vi "MakeProfileMovies.vi"(6 "Plot Metadata":T1[](array[typedef]), 7 "Job Directory":path, 9 "templatePath":path, 10 "Result files to read":path[](array[path]), 11 "suggestedName":string) -> (0 "error out":errorcluster, 3 "automaticFilename":string)   [LabVIEW 2021]
uses:
  Anemometry/Anemometry Sub Vis/Data_plotting_vis/RFP_Plot_Metadata.ctl
  Anemometry/Anemometry Sub Vis/Data_plotting_vis/Error_bars_index.ctl
panel:
  in  "Stop":bool
  out "ffmpegOutput":string
  # "Harvests images corresponding to Raw Data files of plotted series. Joins multiple cam images per measurement, and joins those alongside joined images from other series"
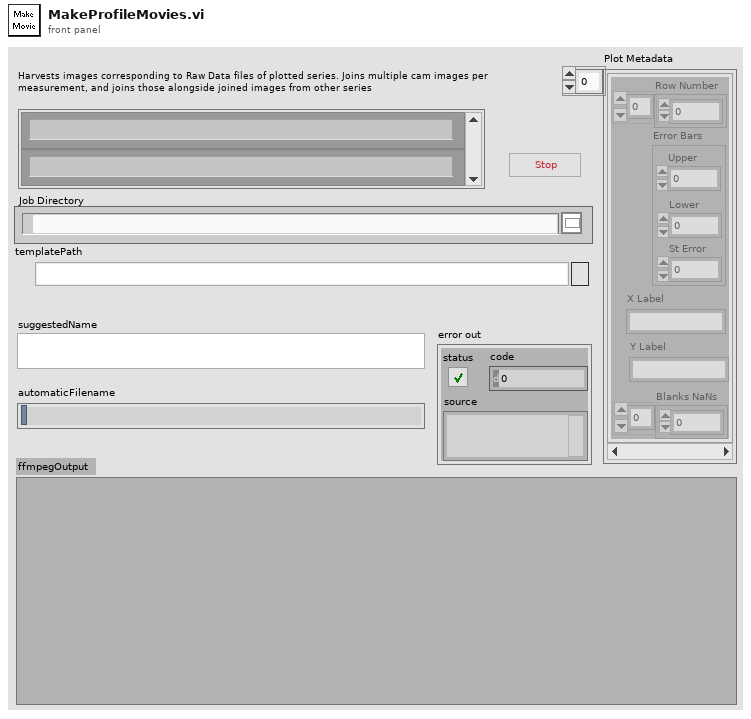
[diagram p1: front panel]
types:
  T1 = typedef "RFP_Plot_Metadata.ctl" = cluster{"Row Number":i32[], "Error Bars":T2, "X Label":string, "Y Label":string, "Blanks NaNs":i32[]}
  T2 = typedef "Error_bars_index.ctl" = cluster{"Upper":i32, "Lower":i32, "St Error":i32}
  T3 = cluster{"new picture":picture, "image path":path}[]
  T4 = typedef "imagedata.ctl" = cluster{"image type":i32, "image depth":i32, "image":u8[], "mask":u8[], "colors":u32[], "Rectangle":cluster{"left":i16, "top":i16, "right":i16, "bottom":i16}}
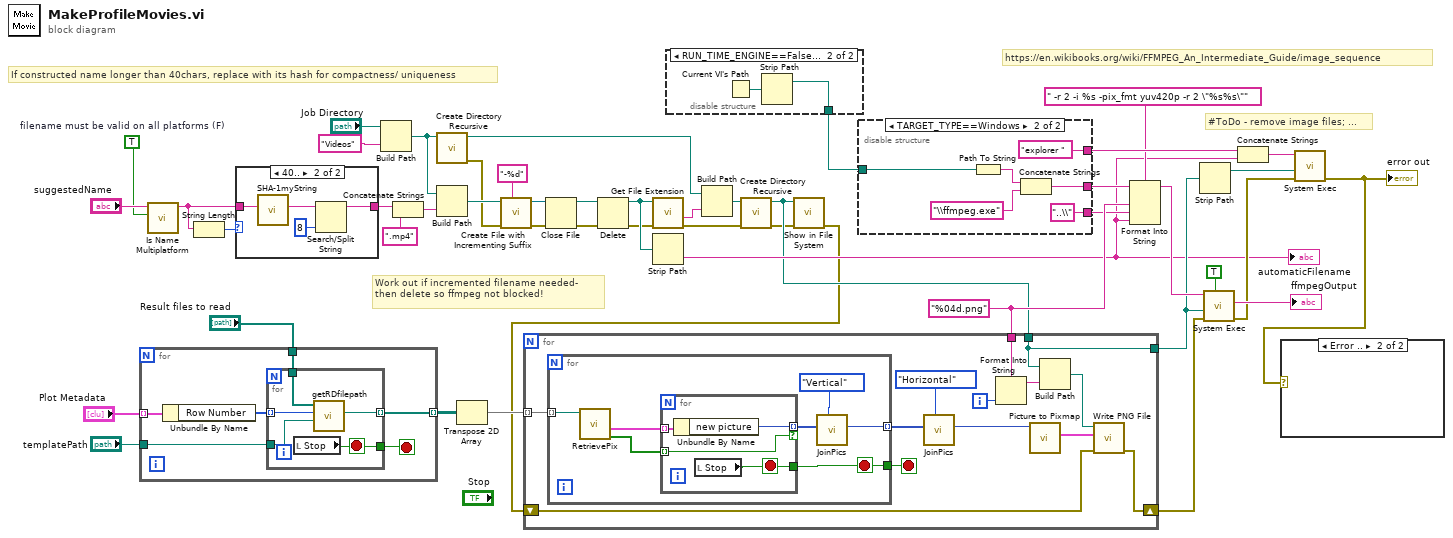
[diagram p0: block diagram]
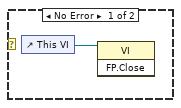
[diagram p2: hidden frame]
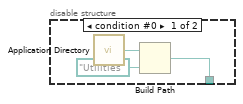
[diagram p3: hidden frame]
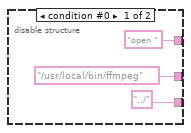
[diagram p5: hidden frame]
diagram:
  w38 = TRUE  # filename must be valid on all platforms (F)
  w27 = "%04d.png" ("format string")
  # "Work out if incremented filename needed- then delete so ffmpeg not blocked!"
  # "If constructed name longer than 40chars, replace with its hash for compactness/ uniqueness"
  # "#ToDo - remove image files; ..."
  # "https://en.wikibooks.org/wiki/FFMPEG_An_Intermediate_Guide/image_sequence"
  n1 = for {
    tunnel: "Plot Metadata" -> [w53] mode=indexing
    tunnel: [w50] -> w45 mode=indexing
    tunnel: "Result files to read" -> [w51]
    tunnel: "templatePath" -> [w49]
    stop <- w48 stop-if-true
    n2 = Unbundle By Name(w53) -> ("Row Number"=w52:i32[])
    n3 = for {
      tunnel: w52 -> [w58] mode=indexing
      tunnel: [w57] -> w50 mode=indexing
      tunnel: w51 -> [w56]
      tunnel: w49 -> [w55]
      tunnel: [w54] -> w48
      stop <- w54 stop-if-true
      n4 = local read "Stop"() -> (w54:bool)
      n5 = call "getRDfilepath.vi"("templatePath"=w55, "rowIndex"=w58, "Result files to read"=w56) -> ("rawDataPath"=w57:path)  [unwired: 6 in, 2 out]
    }
  }
  n6 = call <vilib>:"Is Name Multiplatform.vi"("filename must be valid on all platforms (F)"=w38, "filename"="suggestedName") -> ("suggested filename"=w34:string)  [unwired: 5 in, 4 out]
  n7 = String Length(string=w34) -> (length=w33:i32)
  n8 = case shown="40.." w33 {
    tunnel: w34 -> [w59 w63]
    tunnel: [w59 w60] -> w30
    frame 0, Default {
    }
    frame 40.. {
      n9 = call "SHA-1myString.vi"("HashThis"=w63) -> ("SHA1string"=w62:string)  [unwired: 9 in, 1 out]
      n10 = Search/Split String(string=w62, offset (0)=8) -> (substring before match=w60:string)  [unwired: 1 in, 2 out]
    }
  }
  n11 = Build Path(base path="Job Directory", name or relative path="Videos") -> (appended path=w3:path)
  n12 = Concatenate Strings(w30, ".mp4" ("string")) -> (w21:string)
  n13 = call <vilib>:"Create Directory Recursive.vi"("directory"=w3) -> ("error out"=w1:errorcluster, "directory copy"=w2:path)  [unwired: 4 in, 1 out]
  n14 = Build Path(base path=w3, name or relative path=w21) -> (appended path=w22:path)
  n15 = Transpose 2D Array(2D array=w45) -> (transposed array=w44:path[][])
  n16 = call <vilib>:"Create File with Incrementing Suffix.vi"("format string (\" (%d)\")"="-%d" ("format string (\" (%d)\")"), "error in (no error)"=w1, "file path"=w22) -> ("error out"=w11:errorcluster, "refnum out"=w10:refnum<file>)  [unwired: 6 in, 1 out]
  n17 = Close File(refnum=w10, error in=w11) -> (path=w9:path, error out=w8:errorcluster)
  n18 = Delete(path (use dialog)=w9, error in=w8) -> (deleted path=w16:path, error out=w7:errorcluster)  [unwired: 3 in, 1 out]
  n19 = call <vilib>:"Get File Extension.vi"("error in (no error)"=w7, "file"=w16) -> ("error out"=w13:errorcluster, "filename without extension"=w15:string)  [unwired: 5 in, 3 out]
  n20 = Strip Path(path=w16) -> (name=w20:string)  [unwired: 1 out]
  "automaticFilename" <- w20
  n21 = disable-structure shown="RUN_TIME_ENGINE==False, Default" {
    disable-tunnel: [w64 w67] -> w12
    frame condition #0 {
      n22 = call <vilib>:"Application Directory.vi"() -> ("Application Directory"=w66:path)
      n23 = Build Path(base path=w66, name or relative path=path "Utilities") -> (appended path=w64:path)
    }
    frame condition #1 (active) {
      n24 = Current VI's Path() -> (path=w68:path)
      n25 = Strip Path(path=w68) -> (stripped path=w67:path)  [unwired: 1 out]
    }
  }
  n26 = Build Path(base path=w2, name or relative path=w15) -> (appended path=w19:path)
  n27 = call <vilib>:"Create Directory Recursive.vi"("error in (no error)"=w13, "directory"=w19) -> ("error out"=w17:errorcluster, "directory copy"=w18:path)  [unwired: 3 in, 1 out]
  n28 = call <vilib>:"Show in File System.vi"("error in (no error)"=w17, "file or directory path"=w18) -> ("error out"=w6:errorcluster)  [unwired: 9 in]
  n29 = for {
    tunnel: w44 -> [w81] mode=indexing
    tunnel: w18 -> [w72]
    tunnel: w27 -> [w73]
    tunnel: [w72] -> w23
    shift-right: [w69] -> w5
    shift-left: w6 -> [w70]
    i -> [w74]
    stop <- w71 stop-if-true
    n30 = for {
      tunnel: w81 -> [w88] mode=indexing
      tunnel: [w84] -> w80 mode=indexing
      tunnel: [w82] -> w71
      stop <- w82 stop-if-true
      n31 = call "RetrievePix.vi"("RawDataFile"=w88) -> ("CamSelect"=w83:bool[], "PicPath"=w87:T3)  [unwired: 8 in, 1 out]
      n32 = for {
        tunnel: w87 -> [w92] mode=indexing
        tunnel: [w91] -> w85 mode=indexing if=w90
        tunnel: w83 -> [w90] mode=indexing
        tunnel: [w89] -> w82
        stop <- w89 stop-if-true
        n33 = Unbundle By Name(w92) -> ("new picture"=w91:picture)
        n34 = local read "Stop"() -> (w89:bool)
      }
      n35 = call "JoinPics.vi"("Mode"=enum16{"Horizontal", "Vertical"}."Vertical", "Array-o-pix"=w85) -> ("JoinedPics"=w84:picture)  [unwired: 9 in]
    }
    n36 = call "JoinPics.vi"("Mode"=enum16{"Horizontal", "Vertical"}."Horizontal", "Array-o-pix"=w80) -> ("JoinedPics"=w75:picture)  [unwired: 9 in]
    n37 = Format Into String(format string=w73, w74) -> (resulting string=w77:string)  [unwired: 2 in, 1 out]
    n38 = call <vilib>:"Picture to Pixmap.vi"("picture"=w75) -> ("image data"=w78:T4)  [unwired: 9 in, 1 out]
    n39 = Build Path(base path=w72, name or relative path=w77) -> (appended path=w76:path)
    n40 = call <vilib>:"Write PNG File.vi"("error in (no error)"=w70, "image data"=w78, "path to PNG file"=w76) -> ("error out"=w69:errorcluster)  [unwired: 7 in, 1 out]
  }
  n41 = disable-structure shown="TARGET_TYPE==Windows" {
    disable-tunnel: ["/usr/local/bin/ffmpeg" w101] -> w29
    disable-tunnel: ["open " "explorer "] -> w36
    disable-tunnel: ["../" "..\\"] -> w25
    disable-tunnel: w12 -> [_ w96]
    frame condition #0 {
    }
    frame condition #1 (active) {
      n42 = Path To String(path=w96) -> (string=w100:string)
      n43 = Concatenate Strings(w100, "\\ffmpeg.exe") -> (w101:string)
    }
  }
  n44 = Format Into String(format string=" -r 2 -i %s -pix_fmt yuv420p -r 2 \"%s%s\"", initial string=w29, w27, w25, w20) -> (resulting string=w26:string)  [unwired: 1 in, 1 out]
  n45 = Strip Path(path=w23) -> (stripped path=w24:path)  [unwired: 1 out]
  n46 = call <vilib>:"System Exec.vi"("wait until completion? (T)"=TRUE, "error in (no error)"=w5, "working directory"=w23, "command line"=w26) -> ("error out"=w37:errorcluster, "standard error"=→"ffmpegOutput":string)  [unwired: 4 in, 2 out]
  n47 = Concatenate Strings(w36, w20) -> (w35:string)
  n48 = call <vilib>:"System Exec.vi"("error in (no error)"=w37, "working directory"=w24, "command line"=w35) -> ("error out"=w4:errorcluster)  [unwired: 5 in, 3 out]
  "error out" <- w4
  n49 = case shown="Error .." w4 {
    frame No Error {
      n50 = control-ref of="This VI"() -> (w102:refnum<vi>)
      n51 = invoke class="VI" method="FP.Close"(reference=w102) -> ()  [unwired: 2 in, 3 out]
    }
    frame Error {
    }
  }
